vi "DAQ-AI Mean Value.vi"(10 "clai. Parmeter":T1, 11 "data":dbl[][](array[numeric]) format="%0.2f") -> ()   [LabVIEW 2015]
uses:
  Galobal variable_TI.vi
panel:
  out "AI_as DI":bool[](array[boolean])
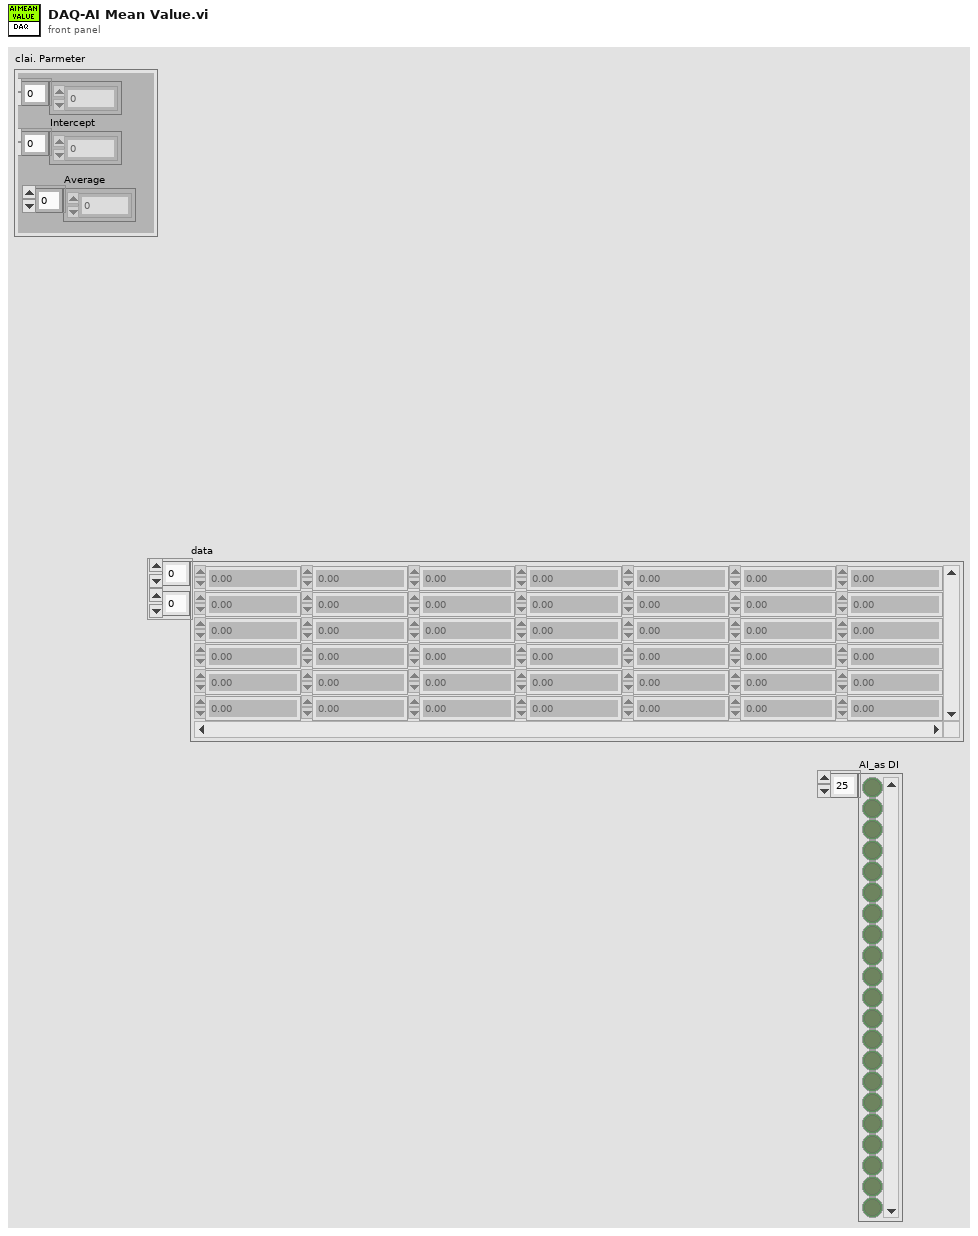
[diagram p1: front panel]
types:
  T1 = cluster{"Slop":dbl[], "Intercept":dbl[], "Average ":i16[]}
  T2 = cluster{"AI-1":dbl, "AI-1 V":dbl, "AI-2":dbl, "AI-2 V":dbl, "AI-3":dbl, "AI- 3v":dbl}
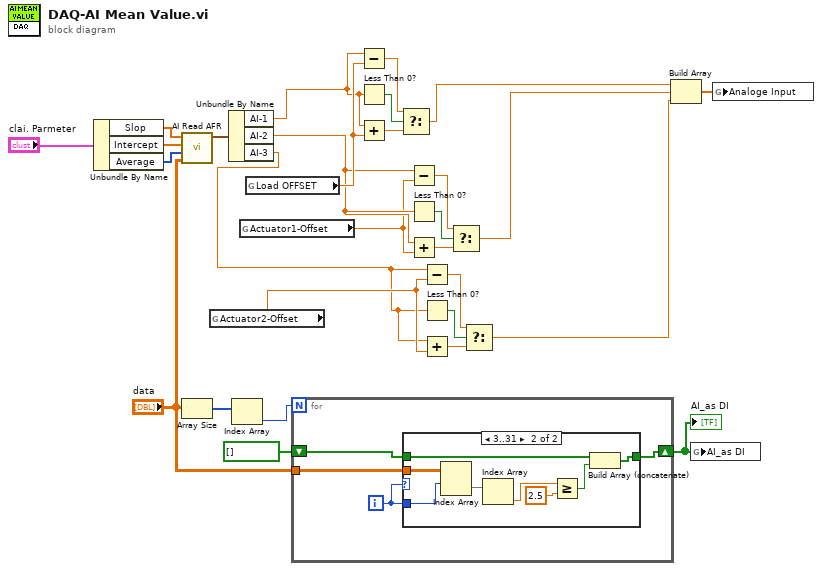
[diagram p0: block diagram]
diagram:
  n1 = Unbundle By Name("clai. Parmeter") -> ("Slop"=w24:dbl[], "Intercept"=w23:dbl[], "Average"=w22:i16[])
  n2 = call "AI Read AFR.vi"("Analog In"="data", "Avg Point"=w22, "Intercept"=w23, "Slope"=w24) -> ("Analog Out"=w20:T2)  [unwired: 7 in]
  n3 = Array Size(array="data") -> (size(s)=w29:i32[])
  n4 = global read "Galobal variable_TI.vi" "Actuator2-Offset"() -> (w3:dbl)
  n5 = Unbundle By Name(w20) -> ("AI-1"=w13:dbl, "AI-2"=w9:dbl, "AI-3"=w2:dbl)
  n6 = Index Array(array=w29) -> (element=w27:i32)  [unwired: 1 in]
  n7 = global read "Galobal variable_TI.vi" "Actuator1-Offset"() -> (w8:dbl)
  n8 = global read "Galobal variable_TI.vi" "Load OFFSET"() -> (w18:dbl)
  n9 = for {
    N: w27 -> [_]
    tunnel: "data" -> [w33]
    shift-right: [w30] -> w26
    shift-left: bool[] [] -> [w31]
    i -> [w32]
    n10 = case shown="3..31" w32 {
      tunnel: w33 -> [_ w42]
      tunnel: w32 -> [_ w40]
      tunnel: [w34 w35] -> w30
      tunnel: w31 -> [w34 w41]
      frame Default {
      }
      frame 3..31 {
        n11 = Index Array(array=w42, index (row)=w40) -> (element=w37:dbl[])  [unwired: 1 in]
        n12 = Index Array(array=w37) -> (element=w39:dbl)  [unwired: 1 in]
        n13 = Greater Or Equal?(x=w39, y=2.5) -> (x >= y?=w36:bool)
        n14 = Build Array (concatenate)(w41, w36) -> (w35:bool[])
      }
    }
  }
  "AI_as DI" <- w26
  n15 = Subtract(x=w13, y=w18) -> (x-y=w17:dbl)
  n16 = Less Than 0?(x=w13) -> (x < 0?=w16:bool)
  n17 = Add(x=w13, y=w18) -> (x+y=w15:dbl)
  n18 = Select(t=w17, s=w16, f=w15) -> (s? t:f=w14:dbl)
  n19 = Subtract(x=w9, y=w8) -> (x-y=w10:dbl)
  n20 = Less Than 0?(x=w9) -> (x < 0?=w11:bool)
  n21 = Add(x=w9, y=w8) -> (x+y=w12:dbl)
  n22 = Subtract(x=w2, y=w3) -> (x-y=w6:dbl)
  n23 = Less Than 0?(x=w2) -> (x < 0?=w5:bool)
  n24 = Add(x=w2, y=w3) -> (x+y=w4:dbl)
  n25 = Select(t=w10, s=w11, f=w12) -> (s? t:f=w7:dbl)
  n26 = Select(t=w6, s=w5, f=w4) -> (s? t:f=w1:dbl)
  n27 = Build Array(w14, w7, w1) -> (w19:dbl[])
  n28 = global write "Galobal variable_TI.vi" "AI_as DI"(w26) -> ()
  n29 = global write "Galobal variable_TI.vi" "Analoge Input"(w19) -> ()
